vi "Select Reference 1.vi"(0 "VOG system":enum16{"Mouse", "Chinchilla"}(ring), 4 "Use Last":bool, 6 "Trigger Edge":i32, 7 "Dir":enum16{"Right", "Left"}(ring), 8 "Posn, Vel, Acc":dbl[][](array[numeric]), 9 "Point2":dbl[][](array[numeric]) format="%.2f", 10 "Point3":dbl[][](array[numeric]) format="%.2f", 11 "Point1":dbl[][](array[numeric]) format="%.2f") -> (1 "Pupil Baseline Info":T1 {"Point3" format="%.2f"; "Point2" format="%.2f"; "Point1" format="%.2f"}, 2 "cancelled":bool, 3 "Radius of eyeball (pixels)":dbl format="%.2f")   [LabVIEW 2016, in "3 dot tracker.lvlib"]
uses:
  3 dot tracker.lvlib
  comm/nan operations/nan operations.lvlib
panel:
  in  "String":string
  in  "Cancel":bool
  out "Valid":bool
  out "Reference":i32
  in  "reference":bool
  out "Targets":dbl[][](graph)
  # "Copyright Americo A. Migliaccio (c) 2002 All Rights Reserved by Author"
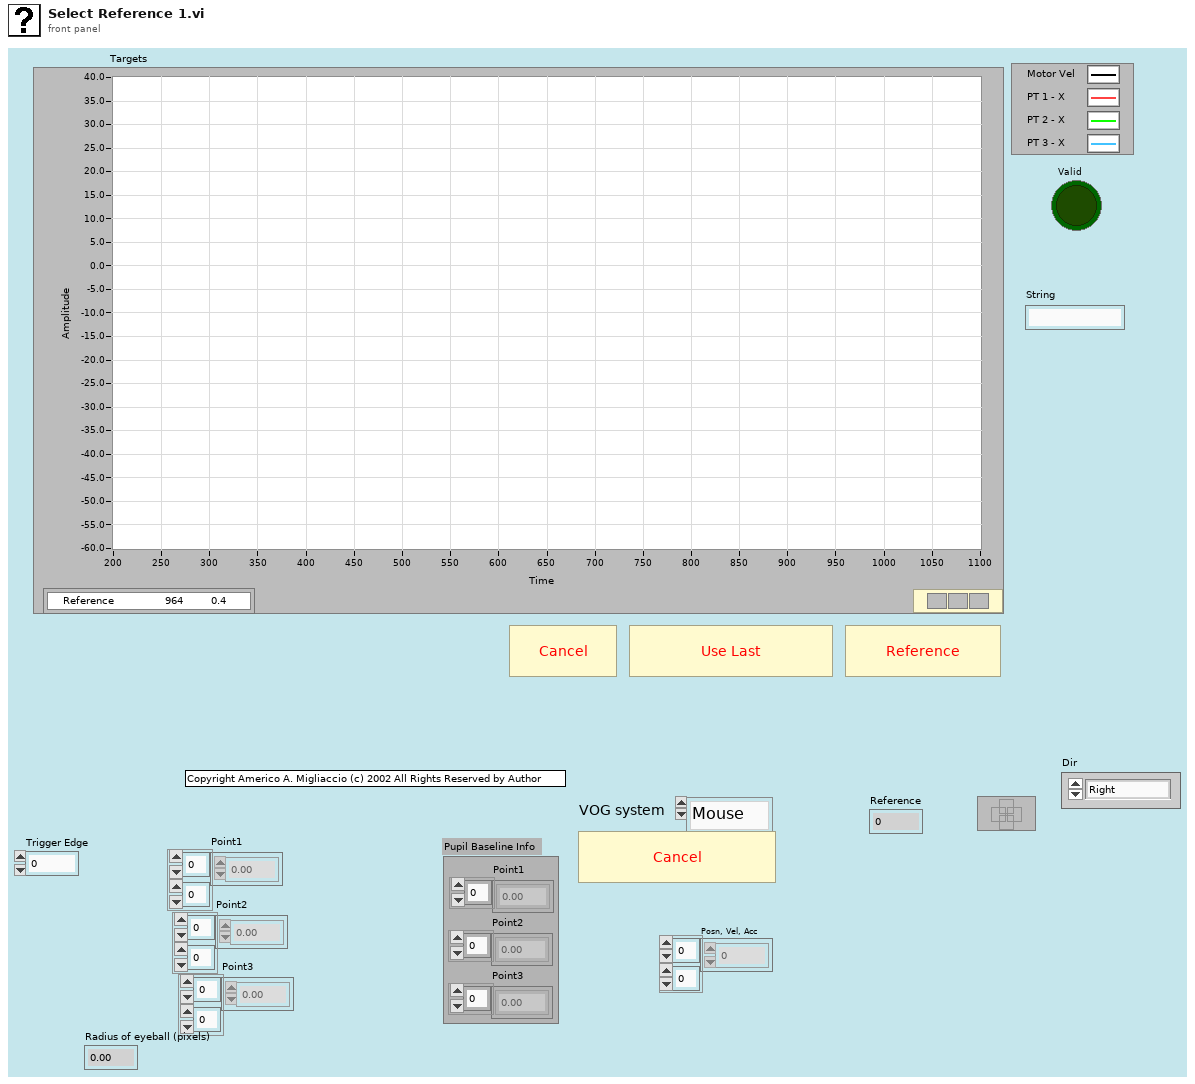
[diagram p1: front panel]
types:
  T1 = cluster{"Point1":dbl[], "Point2":dbl[], "Point3":dbl[]}
  T2 = cluster{"Point1":dbl[], "Point3":dbl[], "Point2":dbl[]}
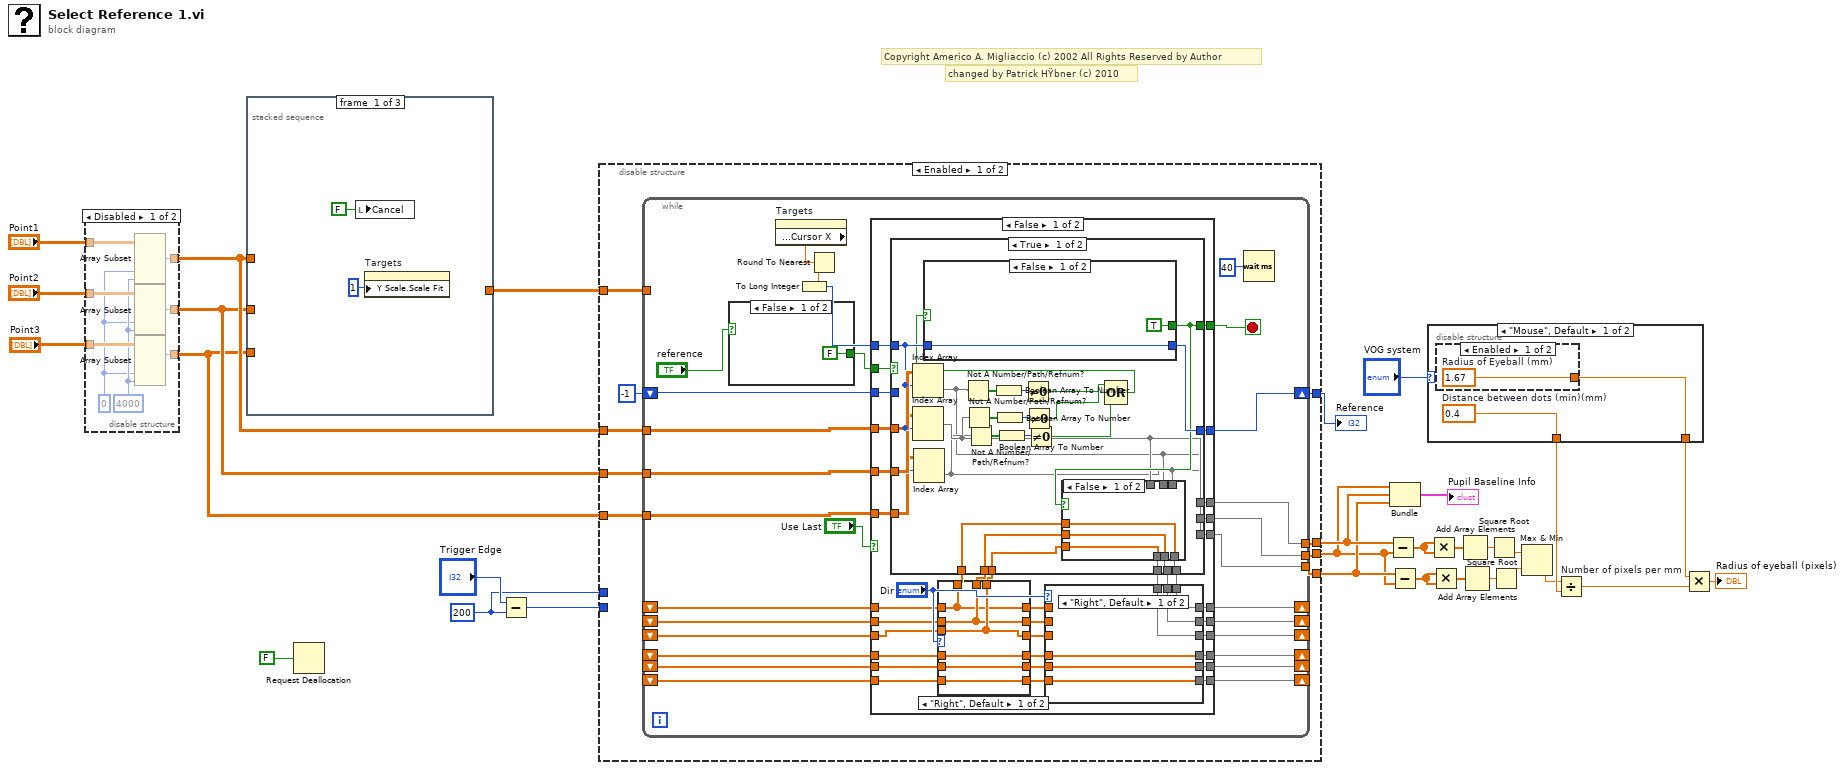
[diagram p0: block diagram]
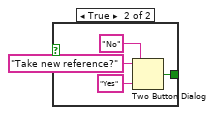
[diagram p3: hidden frame]
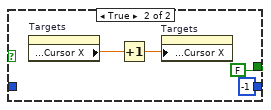
[diagram p7: hidden frame]
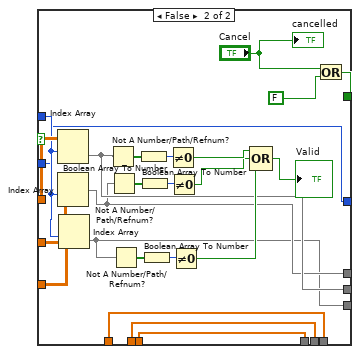
[diagram p8: hidden frame]
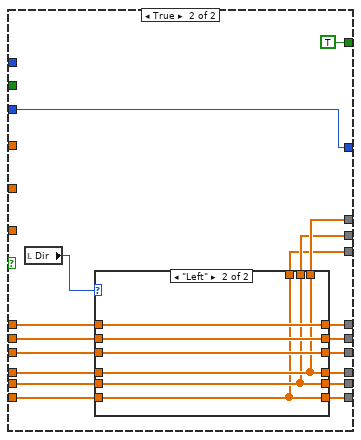
[diagram p9: hidden frame]
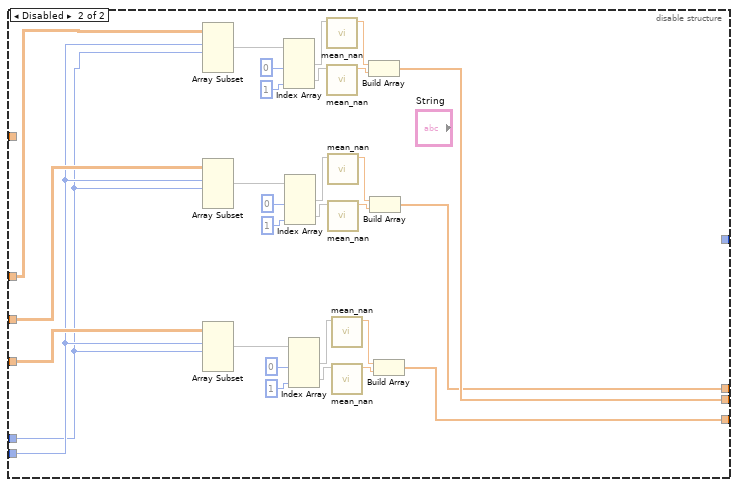
[diagram p11: hidden frame]
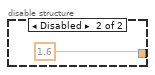
[diagram p12: hidden frame]
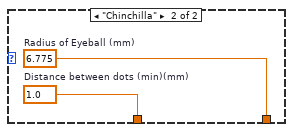
[diagram p13: hidden frame]
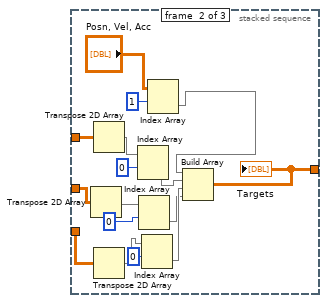
[diagram p14: hidden frame]
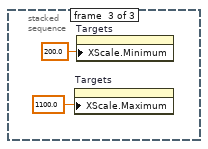
[diagram p15: hidden frame]
diagram:
  w1 = 200
  # "changed by Patrick HŸbner (c) 2010"
  # "Copyright Americo A. Migliaccio (c) 2002 All Rights Reserved by Author"
  n1 = disable-structure shown="Disabled" {
    disable-tunnel: "Point1" -> [w38 w41]
    disable-tunnel: "Point2" -> [w37 w40]
    disable-tunnel: "Point3" -> [w36 w39]
    disable-tunnel: [w33 w41] -> w10
    disable-tunnel: [w32 w40] -> w9
    disable-tunnel: [w31 w39] -> w8
    frame Disabled {
      w35 = 4000 ("length")
      w34 = 0 ("index")
      n2 = Array Subset(array=w38, index (col)=w34, length (col)=w35) -> (w33:dbl[][])  [unwired: 2 in]
      n3 = Array Subset(array=w37, index (col)=w34, length (col)=w35) -> (w32:dbl[][])  [unwired: 2 in]
      n4 = Array Subset(array=w36, index (col)=w34, length (col)=w35) -> (w31:dbl[][])  [unwired: 2 in]
    }
    frame Enabled {
    }
  }
  n5 = stacked-sequence {
    tunnel: [_ w58 _] -> w30
    tunnel: w8 -> [_ w57 _]
    tunnel: w9 -> [_ w47 _]
    tunnel: w10 -> [_ w59 _]
    frame #0 {
      n6 = local write "Cancel"(FALSE ("Cancel")) -> ()
      n7 = property on="Targets" class="WFGraph (strict)"("Y Scale.Scale Fit"=u8 1) -> ()  [unwired: 2 in, 2 out]
    }
    frame #1 {
      n8 = Transpose 2D Array(2D array=w47) -> (transposed array=w46:dbl[][])
      n9 = Transpose 2D Array(2D array=w59) -> (transposed array=w54:dbl[][])
      n10 = Transpose 2D Array(2D array=w57) -> (transposed array=w56:dbl[][])
      n11 = Index Array(array=w54, index (row)=0) -> (element=w53:dbl[])  [unwired: 1 in]
      n12 = Index Array(array=w46, index (row)=0) -> (element=w44:dbl[])  [unwired: 1 in]
      n13 = Index Array(array=w56, index (row)=0) -> (element=w55:dbl[])  [unwired: 1 in]
      n14 = Index Array(array="Posn, Vel, Acc", index (row)=1) -> (element=w51:dbl[])  [unwired: 1 in]
      n15 = Build Array(w51, w53, w55, w44) -> (w58:dbl[][])
      "Targets" <- w58
    }
    frame #2 {
      n16 = property on="Targets" class="WFGraph (strict)"("XScale.Maximum"=1100.0 ("X Scale.Range:Maximum")) -> ()  [unwired: 2 in, 2 out]
      n17 = property on="Targets" class="WFGraph (strict)"("XScale.Minimum"=200.0 ("X Scale.Range:Minimum")) -> ()  [unwired: 2 in, 2 out]
    }
  }
  n18 = Request Deallocation(FALSE ("flag")) -> ()
  n19 = Subtract(x="Trigger Edge", y=w1) -> (x-y=w2:i32)
  n20 = disable-structure shown="Enabled" {
    disable-tunnel: w30 -> [w70 _]
    disable-tunnel: [w68 _] -> w29
    disable-tunnel: w10 -> [w67 w257]
    disable-tunnel: w9 -> [w66 w283]
    disable-tunnel: w8 -> [w65 w282]
    disable-tunnel: [w64 w258] -> w7
    disable-tunnel: [w63 w260] -> w6
    disable-tunnel: [w62 w259] -> w5
    disable-tunnel: w2 -> [_ w256]
    disable-tunnel: w1 -> [_ w255]
    frame Enabled {
      n21 = while {
        shift-left: -1 -> [w88]
        shift-right: [w89] -> w68
        tunnel: w70 -> [_]
        tunnel: w67 -> [w95]
        tunnel: w66 -> [w94]
        tunnel: w65 -> [w93]
        tunnel: [w91] -> w64
        tunnel: [w92] -> w62
        tunnel: [w90] -> w63
        shift-right: [w79] -> _
        shift-left: _ -> [w73]
        shift-right: [w80] -> _
        shift-left: _ -> [w74]
        shift-right: [w81] -> _
        shift-left: _ -> [w75]
        shift-right: [w82] -> _
        shift-left: _ -> [w76]
        shift-right: [w83] -> _
        shift-left: _ -> [w77]
        shift-right: [w84] -> _
        shift-left: _ -> [w78]
        stop <- w86 stop-if-true
        n22 = case shown="False" "reference" {
          tunnel: [FALSE ("T button?") w100] -> w71
          frame False {
          }
          frame True {
            n23 = Two Button Dialog(message="Take new reference?", 1:"No" ("F button name (\"Cancel\")"), 2:"Yes" ("T button name (\"OK\")")) -> (T button?=w100:bool)
          }
        }
        n24 = property on="Targets" class="WFGraph (strict)"() -> ("Cursor.Cursor Position:Cursor X"=w98:dbl)  [unwired: 2 in, 2 out]
        n25 = Round To Nearest(number=w98) -> (nearest integer value=w97:dbl)
        n26 = To Long Integer(number=w97) -> (32bit integer=w87:i32)
        n27 = case shown="False" "Use Last" {
          tunnel: w95 -> [w139 _]
          tunnel: w94 -> [w138 _]
          tunnel: w93 -> [w137 _]
          tunnel: [w136 w226] -> w92
          tunnel: [w135 w227] -> w91
          tunnel: [w134 w225] -> w90
          tunnel: [w133 w242] -> w89
          tunnel: w71 -> [w132 _]
          tunnel: w88 -> [w131 w242]
          tunnel: w87 -> [w130 _]
          tunnel: [w129 TRUE] -> w86
          tunnel: [w125 w238] -> w84
          tunnel: [w124 w236] -> w83
          tunnel: [w123 w234] -> w82
          tunnel: [w122 w232] -> w81
          tunnel: [w121 w230] -> w80
          tunnel: [w120 w228] -> w79
          tunnel: w78 -> [w108 w239]
          tunnel: w77 -> [w109 w237]
          tunnel: w76 -> [w112 w235]
          tunnel: w75 -> [w113 w233]
          tunnel: w74 -> [w116 w231]
          tunnel: w73 -> [w118 w229]
          frame False {
            n28 = case shown="\"Right\", Default" "Dir" {
              tunnel: w118 -> [w140 w146]
              tunnel: [w140 w146] -> w117
              tunnel: w116 -> [w141 w147]
              tunnel: [w141 w147] -> w115
              tunnel: [w142 w148] -> w114
              tunnel: w113 -> [w142 w148]
              tunnel: w112 -> [w145 w151]
              tunnel: [w145 w151] -> w111
              tunnel: [w144 w150] -> w110
              tunnel: w109 -> [w144 w150]
              tunnel: w108 -> [w143 w149]
              tunnel: [w143 w149] -> w107
              tunnel: [w143 w148] -> w106
              tunnel: [w144 w147] -> w105
              tunnel: [w145 w146] -> w104
              frame "Right", Default {
              }
              frame "Left" {
              }
            }
            n29 = case shown="True" w132 {
              tunnel: [w184 w207] -> w133
              tunnel: w139 -> [w188 w214]
              tunnel: w138 -> [w187 w213]
              tunnel: w137 -> [w186 w212]
              tunnel: [w168 w210] -> w136
              tunnel: [w172 w209] -> w135
              tunnel: [w170 w208] -> w134
              tunnel: w131 -> [_ w207]
              tunnel: w130 -> [w185 w211]
              tunnel: [w173 w206] -> w129
              tunnel: [w169 w201] -> w128
              tunnel: [w167 w202] -> w127
              tunnel: [w171 w203] -> w126
              tunnel: w104 -> [w166 w203]
              tunnel: w105 -> [w165 w202]
              tunnel: w106 -> [w164 w201]
              frame True {
                n30 = Index Array(array=w188, index (row)=w185) -> (element=w168:dbl[])  [unwired: 1 in]
                n31 = Index Array(array=w187, index (row)=w185) -> (element=w172:dbl[])  [unwired: 1 in]
                n32 = Index Array(array=w186, index (row)=w185) -> (element=w170:dbl[])  [unwired: 1 in]
                n33 = Not A Number/Path/Refnum?(number/path/refnum=w168) -> (NaN/Path/Refnum?=w183:bool[])
                n34 = Not A Number/Path/Refnum?(number/path/refnum=w172) -> (NaN/Path/Refnum?=w180:bool[])
                n35 = Not A Number/Path/Refnum?(number/path/refnum=w170) -> (NaN/Path/Refnum?=w179:bool[])
                n36 = Boolean Array To Number(Boolean array=w183) -> (number=w182:u32)
                n37 = Boolean Array To Number(Boolean array=w180) -> (number=w181:u32)
                n38 = Boolean Array To Number(Boolean array=w179) -> (number=w178:u32)
                n39 = Not Equal To 0?(x=w182) -> (x != 0?=w177:bool)
                n40 = Not Equal To 0?(x=w181) -> (x != 0?=w176:bool)
                n41 = Not Equal To 0?(x=w178) -> (x != 0?=w175:bool)
                n42 = Compound Arithmetic op=OR(w177, w176, w175) -> (w174:bool)
                n43 = case shown="False" w174 {
                  tunnel: [w196 -1] -> w184
                  tunnel: w185 -> [w196 _]
                  tunnel: [TRUE FALSE] -> w173
                  frame False {
                  }
                  frame True {
                    n44 = property on="Targets" class="WFGraph (strict)"() -> ("Cursor.Cursor Position:Cursor X"=w199:dbl)  [unwired: 2 in, 2 out]
                    n45 = Increment(x=w199) -> (x+1=w200:dbl)
                    n46 = property on="Targets" class="WFGraph (strict)"("Cursor.Cursor Position:Cursor X"=w200) -> ()  [unwired: 2 in, 2 out]
                  }
                }
                n47 = case shown="False" w173 {
                  tunnel: w172 -> [_ w194]
                  tunnel: [w191 w194] -> w171
                  tunnel: w170 -> [_ w193]
                  tunnel: [w189 w193] -> w169
                  tunnel: w168 -> [_ w192]
                  tunnel: [w190 w192] -> w167
                  tunnel: w166 -> [w191 _]
                  tunnel: w165 -> [w190 _]
                  tunnel: w164 -> [w189 _]
                  frame False {
                  }
                  frame True {
                  }
                }
              }
              frame False {
                n48 = Index Array(array=w214, index (row)=w211) -> (element=w210:dbl[])  [unwired: 1 in]
                n49 = Index Array(array=w213, index (row)=w211) -> (element=w209:dbl[])  [unwired: 1 in]
                n50 = Index Array(array=w212, index (row)=w211) -> (element=w208:dbl[])  [unwired: 1 in]
                n51 = Not A Number/Path/Refnum?(number/path/refnum=w210) -> (NaN/Path/Refnum?=w224:bool[])
                n52 = Not A Number/Path/Refnum?(number/path/refnum=w209) -> (NaN/Path/Refnum?=w221:bool[])
                n53 = Not A Number/Path/Refnum?(number/path/refnum=w208) -> (NaN/Path/Refnum?=w220:bool[])
                n54 = Boolean Array To Number(Boolean array=w224) -> (number=w223:u32)
                n55 = Boolean Array To Number(Boolean array=w221) -> (number=w222:u32)
                n56 = Boolean Array To Number(Boolean array=w220) -> (number=w219:u32)
                n57 = Not Equal To 0?(x=w223) -> (x != 0?=w218:bool)
                n58 = Not Equal To 0?(x=w222) -> (x != 0?=w217:bool)
                n59 = Not Equal To 0?(x=w219) -> (x != 0?=w216:bool)
                n60 = Compound Arithmetic op=OR(w218, w217, w216) -> (→"Valid":bool)
                n61 = Or(x="Cancel", y=FALSE) -> (x .or. y?=w206:bool)
                "cancelled" <- "Cancel"
              }
            }
            n62 = case shown="\"Right\", Default" "Dir" {
              tunnel: [w157 w160] -> w125
              tunnel: w128 -> [w157 w163]
              tunnel: [w156 w159] -> w124
              tunnel: w127 -> [w156 w162]
              tunnel: [w155 w158] -> w123
              tunnel: w126 -> [w155 w161]
              tunnel: [w154 w163] -> w122
              tunnel: [w153 w162] -> w121
              tunnel: [w152 w161] -> w120
              tunnel: w107 -> [_ w160]
              tunnel: w110 -> [_ w159]
              tunnel: w111 -> [_ w158]
              tunnel: w114 -> [w154 _]
              tunnel: w115 -> [w153 _]
              tunnel: w117 -> [w152 _]
              frame "Right", Default {
              }
              frame "Left" {
              }
            }
          }
          frame True {
            n63 = local read "Dir"() -> (w240:enum16{"Right", "Left"})
            n64 = case shown="\"Left\"" w240 {
              tunnel: w239 -> [w245 w254]
              tunnel: [w245 w254] -> w238
              tunnel: w237 -> [w243 w253]
              tunnel: [w243 w253] -> w236
              tunnel: w235 -> [w244 w252]
              tunnel: [w244 w252] -> w234
              tunnel: w233 -> [w248 w251]
              tunnel: [w248 w251] -> w232
              tunnel: w231 -> [w247 w250]
              tunnel: [w247 w250] -> w230
              tunnel: w229 -> [w246 w249]
              tunnel: [w246 w249] -> w228
              tunnel: [w245 w251] -> w227
              tunnel: [w243 w250] -> w226
              tunnel: [w244 w249] -> w225
              frame "Right", Default {
              }
              frame "Left" {
              }
            }
          }
        }
        n65 = Wait (ms)(milliseconds to wait=u32 40) -> ()  [unwired: 1 out]
      }
    }
    frame Disabled {
      n66 = Array Subset(array=w257, index (row)=w256, length (row)=w255) -> (w281:dbl[][])  [unwired: 2 in]
      n67 = Array Subset(array=w283, index (row)=w256, length (row)=w255) -> (w268:dbl[][])  [unwired: 2 in]
      n68 = Array Subset(array=w282, index (row)=w256, length (row)=w255) -> (w261:dbl[][])  [unwired: 2 in]
      n69 = Index Array(array=w281, index (col) #1=0 ("disabled index (col)"), index (col) #2=1 ("index (col)")) -> (element #1=w278:dbl[], element #2=w277:dbl[])  [unwired: 2 in]
      n70 = Index Array(array=w268, index (col) #1=0 ("disabled index (col)"), index (col) #2=1 ("index (col)")) -> (element #1=w271:dbl[], element #2=w272:dbl[])  [unwired: 2 in]
      n71 = Index Array(array=w261, index (col) #1=0 ("disabled index (col)"), index (col) #2=1 ("index (col)")) -> (element #1=w265:dbl[], element #2=w264:dbl[])  [unwired: 2 in]
      n72 = call "mean_nan.vi"("Array"=w278) -> ("Mean"=w276:dbl)  [unwired: 10 in]
      n73 = call "mean_nan.vi"("Array"=w277) -> ("Mean"=w275:dbl)  [unwired: 10 in]
      n74 = call "mean_nan.vi"("Array"=w271) -> ("Mean"=w273:dbl)  [unwired: 10 in]
      n75 = call "mean_nan.vi"("Array"=w272) -> ("Mean"=w274:dbl)  [unwired: 10 in]
      n76 = call "mean_nan.vi"("Array"=w265) -> ("Mean"=w263:dbl)  [unwired: 10 in]
      n77 = call "mean_nan.vi"("Array"=w264) -> ("Mean"=w262:dbl)  [unwired: 10 in]
      n78 = Build Array(w276, w275) -> (w259:dbl[])
      n79 = Build Array(w273, w274) -> (w258:dbl[])
      n80 = Build Array(w263, w262) -> (w260:dbl[])
    }
  }
  "Reference" <- w29
  n81 = Subtract(x=w7, y=w5) -> (x-y=w20:dbl[])
  n82 = Bundle("Point1"=w5, "Point3"=w7, "Point2"=w6) -> (→"Pupil Baseline Info":T2)  [unwired: 1 in]
  n83 = Subtract(x=w6, y=w5) -> (x-y=w21:dbl[])
  n84 = case shown="\"Mouse\", Default" "VOG system" {
    tunnel: [w284 w289] -> w17
    tunnel: [w285 w288] -> w14
    frame "Mouse", Default {
      w284 = 0.4  # Distance between dots (min)(mm)
      n85 = disable-structure shown="Enabled" {
        disable-tunnel: [w286 1.6] -> w285
        frame Enabled {
          w286 = 1.67  # Radius of Eyeball (mm)
        }
        frame Disabled {
        }
      }
    }
    frame "Chinchilla" {
      w289 = 1.0  # Distance between dots (min)(mm)
      w288 = 6.775  # Radius of Eyeball (mm)
    }
  }
  n86 = Multiply(x=w20, y=w20) -> (x*y=w25:dbl[])
  n87 = Multiply(x=w21, y=w21) -> (x*y=w22:dbl[])
  n88 = Add Array Elements(numeric array=w25) -> (sum=w24:dbl)
  n89 = Add Array Elements(numeric array=w22) -> (sum=w23:dbl)
  n90 = Square Root(x=w24) -> (sqrt(x)=w18:dbl)
  n91 = Square Root(x=w23) -> (sqrt(x)=w19:dbl)
  n92 = Max & Min(x=w18, y=w19) -> (min(x,y)=w16:dbl)  [unwired: 1 out]
  n93 = Divide "Number of pixels per mm"(x=w16, y=w17) -> (x/y=w15:dbl)
  n94 = Multiply(x=w14, y=w15) -> (x*y=→"Radius of eyeball (pixels)":dbl)
